vi "New_group_menu.vi"(8 "error in (no error)":errorcluster, 11 "Default Name":string) -> (0 "error out":errorcluster, 3 "Group Name":string)   [LabVIEW 2013]
doc: "Allows the user to create a new group in the database."
uses:
  <vilib>/Utility/miscctls.llb/LVPointTypeDef.ctl
  <vilib>/Utility/error.llb/DialogType.ctl
  Sub-Polymorphic/post_new_group.vi
  <vilib>/addons/database/_DB Variant To Data/Database Variant To Data.xnode
panel:
  in  "All Groups":string[](array[string])
  in  "Cancel":bool
  in  "New Entry":bool caption="OK2"
  in  "Group Name:":string
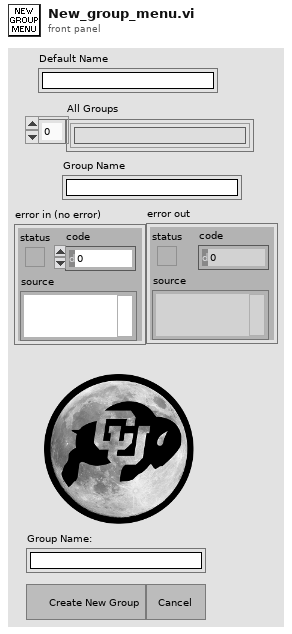
[diagram p1: front panel]
types:
  T1 = typedef "LVPointTypeDef.ctl" = cluster{"Horizontal":i16, "Vertical":i16}
  T2 = typedef "DialogType.ctl" = u16
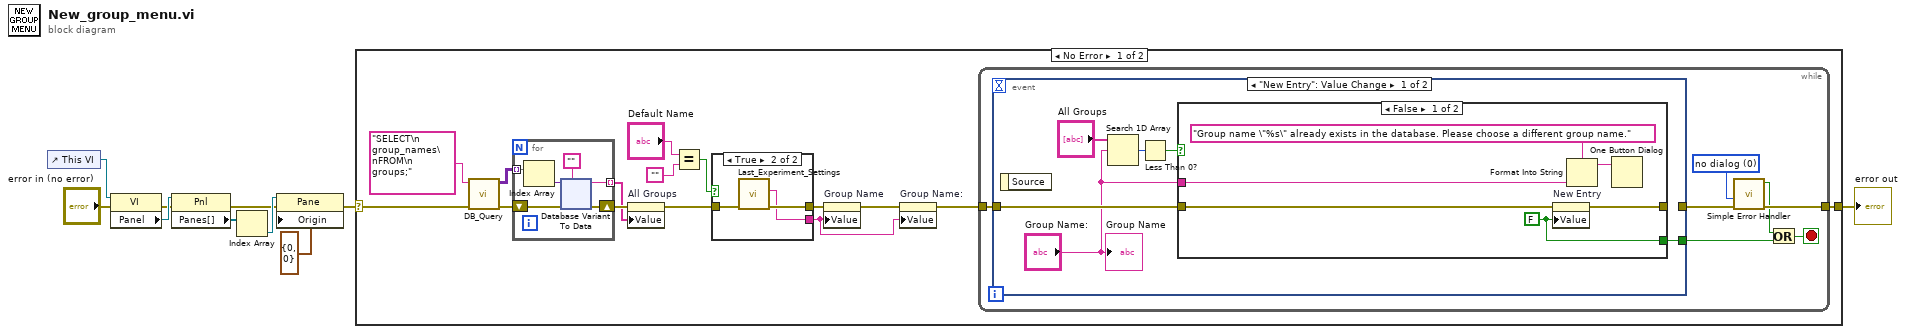
[diagram p0: block diagram]
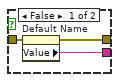
[diagram p2: hidden frame]
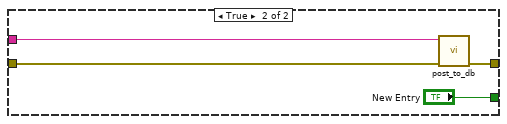
[diagram p3: hidden frame]
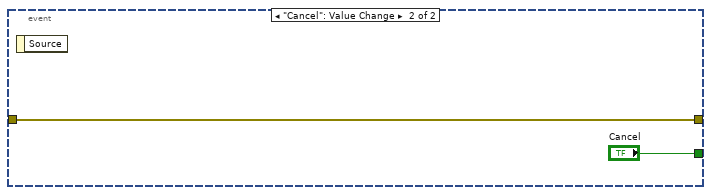
[diagram p4: hidden frame]
diagram:
  n1 = control-ref of="This VI"() -> (w3:refnum<vi>)
  n2 = property class="VI"(reference=w3, error in="error in (no error)") -> (error out=w4:errorcluster, "Panel"=w5:refnum<vi>)  [unwired: 1 out]
  n3 = property class="Pnl"(reference=w5, error in=w4) -> (error out=w6:errorcluster, "Panes[]"=w7:refnum<vi>[])  [unwired: 1 out]
  n4 = Index Array(array=w7) -> (element=w8:refnum<vi>)  [unwired: 1 in]
  n5 = property class="Pane"(reference=w8, error in=w6, "Origin"=T1 {"Horizontal"=0, "Vertical"=0}) -> (error out=w1:errorcluster)  [unwired: 1 out]
  n6 = case shown="No Error" w1 {
    selector: w1 -> [w19 w95]
    tunnel: [w24 w95] -> w10
    frame No Error {
      n7 = call "DB_Query.vi"("error in (no error)"=w19, "Parameterized Query"="SELECT\n  group_names\nFROM\n  groups;") -> ("error out"=w17:errorcluster, "Results"=w15:variant[][])  [unwired: 7 in, 1 out]
      n8 = for {
        shift-right: [w37] -> w18
        shift-left: w17 -> [w36]
        tunnel: w15 -> [w33] mode=indexing
        tunnel: [w32] -> w14 mode=indexing
        n9 = Index Array(array=w33) -> (element=w34:variant)  [unwired: 1 in]
        n10 = xnode "Database Variant To Data"("database variant"=w34, "error in (no error)"=w36, "type"="") -> ("data"=w32:string, "error out"=w37:errorcluster)
      }
      n11 = property on="All Groups" class="Arr (strict)"(error in=w18, "Value"=w14) -> (error out=w20:errorcluster)  [unwired: 1 in, 1 out]
      n12 = Equal?(x="Default Name", y="") -> (x = y?=w11:bool)
      n13 = case shown="True" w11 {
        tunnel: [w28 w31] -> w25
        tunnel: [w27 w30] -> w21
        tunnel: w20 -> [w26 w29]
        frame False {
          n14 = property on="Default Name" class="Str"(error in=w26) -> (error out=w28:errorcluster, "Value"=w27:string)  [unwired: 1 in, 1 out]
        }
        frame True {
          n15 = call "Last_Experiment_Settings.vi"("error in (no error)"=w29) -> ("error out"=w31:errorcluster, "Group Name"=w30:string)  [unwired: 5 in, 4 out]
        }
      }
      n16 = property on="Group Name" class="Str"(error in=w25, "Value"=w21) -> (error out=w23:errorcluster)  [unwired: 1 in, 1 out]
      n17 = property on="Group Name:" class="Str"(error in=w23, "Value"=w21) -> (error out=w22:errorcluster)  [unwired: 1 in, 1 out]
      n18 = while {
        tunnel: [w74] -> w24
        tunnel: w22 -> [w75]
        stop <- w71 stop-if-true
        w70 = T2 0 items=["no dialog", "OK message", "continue or stop message", "OK message + warnings", "continue/stop + warnings"] ("type of dialog (OK msg:1)")
        n19 = event shown="[0] \"New Entry\": Value Change" {
          selector: _ -> [_ _]
          dyn-events: _ -> [_ _]
          timeout: _ -> [_ _]
          tunnel: w75 -> [w81 w94]
          tunnel: [_ w94] -> w76
          tunnel: [w82 "Cancel"] -> w72
          event "New Entry": Value Change {
            n20 = event-data() -> ()  [unwired: 1 in, 1 out]
            n21 = Search 1D Array(1D array="All Groups", element="Group Name:") -> (index of element=w78:i32)  [unwired: 1 in]
            n22 = Less Than 0?(x=w78) -> (x < 0?=w77:bool)
            n23 = case shown="False" w77 {
              tunnel: [w84 w92] -> _
              tunnel: [w83 "New Entry"] -> w82
              tunnel: w81 -> [w85 w90]
              tunnel: "Group Name:" -> [w86 w89]
              frame False {
                w83 = FALSE ("New Entry")
                n24 = property on="New Entry" class="Bool (strict)"(error in=w85, "Value"=w83) -> (error out=w84:errorcluster)  [unwired: 1 in, 1 out]
                n25 = Format Into String(format string="Group name \"%s\" already exists in the database. Please choose a different group name.", w86) -> (resulting string=w87:string)  [unwired: 2 in, 1 out]
                n26 = One Button Dialog(message=w87) -> ()  [unwired: 1 in, 1 out]
              }
              frame True {
                n27 = call-poly "post_to_db.vi"("error in (no error)"=w90, "Group Name"=w89) -> ("error out"=w92:errorcluster)  [unwired: 9 in]
              }
            }
            "Group Name" <- "Group Name:"
          }
          event "Cancel": Value Change {
            n28 = event-data() -> ()  [unwired: 1 in, 1 out]
          }
        }
        n29 = call <vilib>:"Simple Error Handler.vi"("type of dialog (OK msg:1)"=w70, "error in (no error)"=w76) -> ("error?"=w73:bool, "error out"=w74:errorcluster)  [unwired: 3 in, 3 out]
        n30 = Or(x=w73, y=w72) -> (x .or. y?=w71:bool)
      }
    }
    frame Error {
    }
  }
  "error out" <- w10
